vi "Multiply Waveform By Signal.vi"(1 "Signal in":dbl[](array[numeric]), 2 "Waveform in":waveform(dbl)) -> (0 "Waveform out":waveform(dbl))   [LabVIEW 2019]
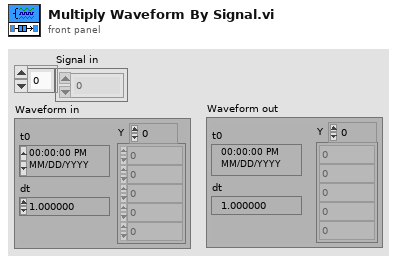
[diagram p1: front panel]
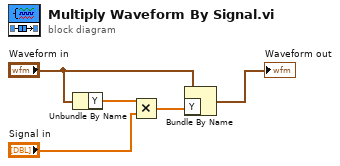
[diagram p0: block diagram]
diagram:
  n1 = Unbundle By Name("Waveform in") -> ("Y"=w2:dbl[])
  n2 = Multiply(x=w2, y="Signal in") -> (x*y=w5:dbl[])
  n3 = Bundle By Name(cluster="Waveform in", "Y"=w5) -> (→"Waveform out":waveform(dbl))
